vi "Filter_2D_array.vi"(0 "All 2D data":dbl[][](array[numeric]) format="%.3f", 3 "Accept array":bool[](array[boolean])) -> (5 "Filtered data":dbl[][](array[numeric]) format="%.3f", 6 "No of points removed":i32)   [LabVIEW 2010]
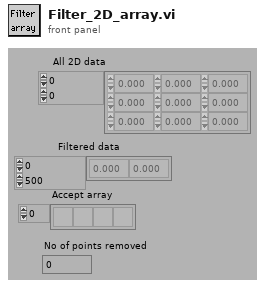
[diagram p1: front panel]
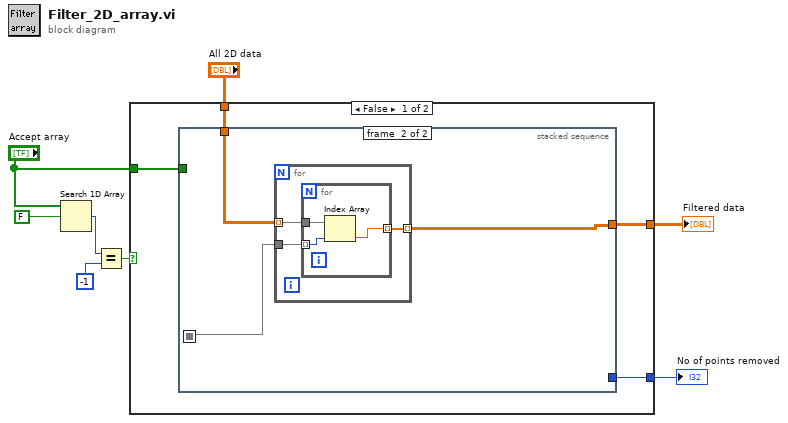
[diagram p0: block diagram]
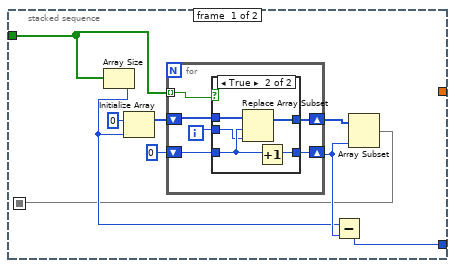
[diagram p2: hidden frame]
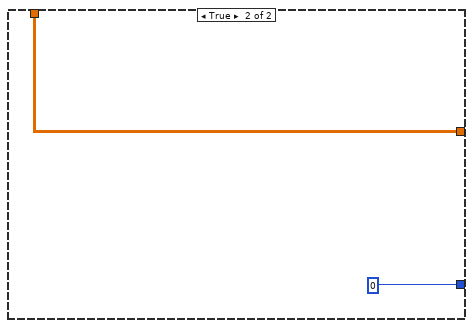
[diagram p4: hidden frame]
diagram:
  n1 = Search 1D Array(1D array="Accept array", element=FALSE) -> (index of element=w3:i32)  [unwired: 1 out]
  n2 = Equal?(x=w3, y=-1) -> (x = y?=w2:bool)
  n3 = case shown="False" w2 {
    tunnel: "All 2D data" -> [w12 w45]
    tunnel: "Accept array" -> [w11 _]
    tunnel: [w10 w45] -> w7
    tunnel: [w9 0] -> w8
    frame False {
      n4 = stacked-sequence {
        seq-local: [w13 _] -> [_ w37]
        tunnel: w12 -> [_ w36]
        tunnel: w11 -> [w15 _]
        tunnel: [_ w35] -> w10
        tunnel: [w14 _] -> w9
        frame #0 {
          n5 = Array Size(array=w15) -> (size(s)=w20:i32)
          n6 = Initialize Array(0, w20) -> (w18:i32[])
          n7 = for {
            shift-right: [w25] -> w16
            shift-left: w18 -> [w26]
            tunnel: w15 -> [w27] mode=indexing
            shift-right: [w23] -> w21
            shift-left: 0 -> [w24]
            i -> [w22]
            n8 = case shown="True" w27 {
              tunnel: w26 -> [w29 w34]
              tunnel: [w29 w33] -> w25
              tunnel: w24 -> [w28 w32]
              tunnel: [w28 w31] -> w23
              tunnel: w22 -> [_ w30]
              frame False {
              }
              frame True {
                n9 = Replace Array Subset(array=w34, new element=w30, index=w32) -> (w33:i32[])
                n10 = Increment(x=w32) -> (x+1=w31:i32)
              }
            }
          }
          n11 = Subtract(x=w20, y=w21) -> (x-y=w14:i32)
          n12 = Array Subset(array=w16, length=w21) -> (w13:i32[])  [unwired: 1 in]
        }
        frame #1 {
          n13 = for {
            tunnel: w36 -> [w40] mode=indexing
            tunnel: w37 -> [w39]
            tunnel: [w38] -> w35 mode=indexing
            n14 = for {
              tunnel: w39 -> [w42] mode=indexing
              tunnel: w40 -> [w43]
              tunnel: [w41] -> w38 mode=indexing
              n15 = Index Array(array=w43, index=w42) -> (element=w41:dbl)
            }
          }
        }
      }
    }
    frame True {
    }
  }
  "Filtered data" <- w7
  "No of points removed" <- w8
